vi "C3 to Cube and Switch.vi"(8 "Command Info In":T1, 10 "Block Inputs":T5, 11 "Starting Position":T4) -> (0 "Command Info Out":T1)   [LabVIEW 2017]
uses:
  <vilib>/Rock Robotics/WPI/Framework/Command Status Info.ctl
  <vilib>/Rock Robotics/WPI/Framework/Completion Status.ctl
  <vilib>/Rock Robotics/WPI/Framework/Completion Notifier.ctl
  Block Clusters/C3 to Cube and Switch.ctl
  Support Code/Starting Position.ctl
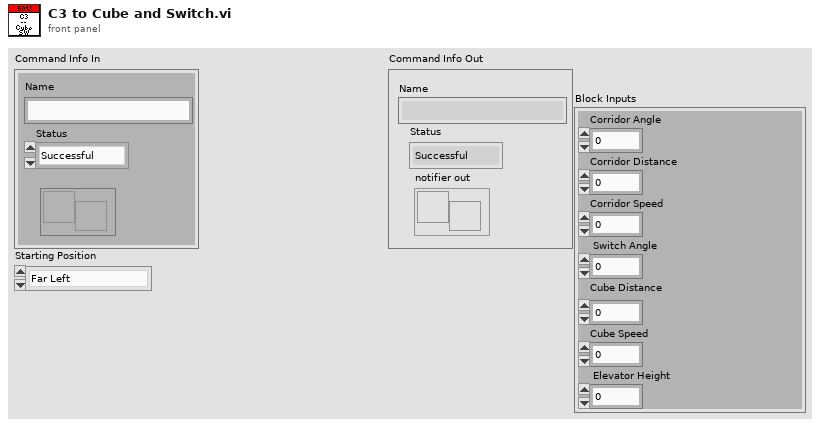
[diagram p1: front panel]
types:
  T1 = typedef "Command Status Info.ctl" = cluster{"Name":string, "Status":T2, "notifier out":T3}
  T2 = typedef "Completion Status.ctl" = enum16{"Successful", "Aborted", "Incomplete"}
  T3 = typedef "Completion Notifier.ctl" = refnum<notifier>
  T4 = typedef "Starting Position.ctl" = enum16{"Far Left", "Center", "Far Right"}
  T5 = typedef "C3 to Cube and Switch.ctl" = cluster{"Corridor Angle":dbl, "Corridor Distance":dbl, "Corridor Speed":dbl, " Switch Angle":dbl, "Cube Distance":dbl, "Cube Speed":dbl, " Elevator Height":dbl}
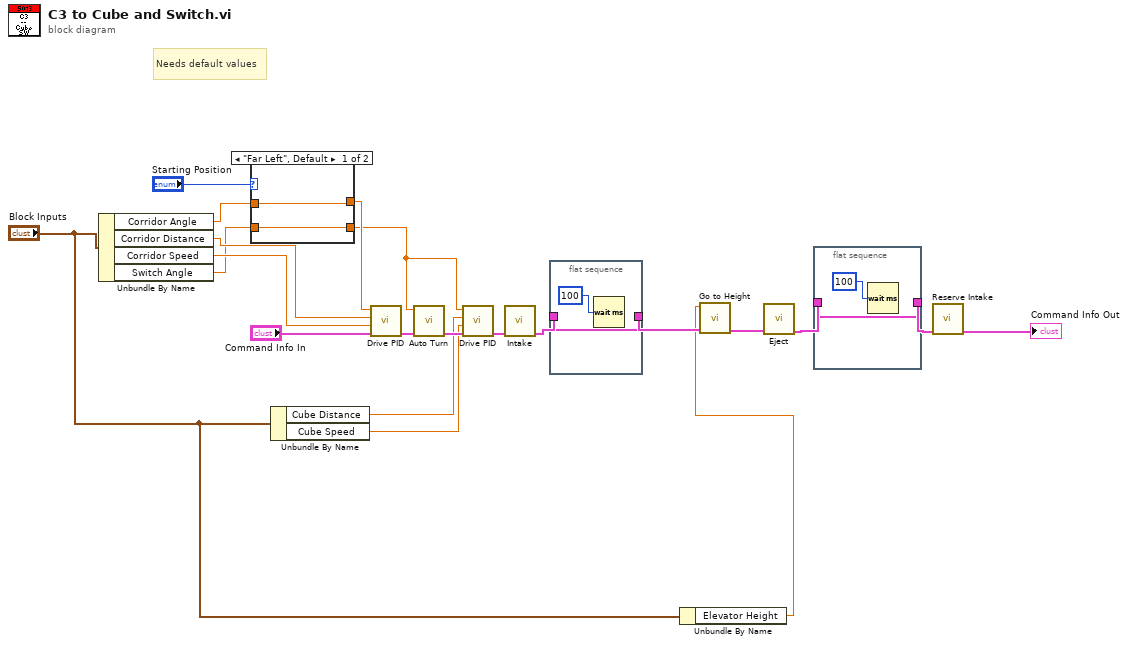
[diagram p0: block diagram]
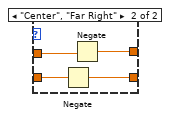
[diagram p2: hidden frame]
diagram:
  # "Needs default values"
  n1 = Unbundle By Name("Block Inputs") -> ("Corridor Angle"=w10:dbl, "Corridor Distance"=w8:dbl, "Corridor Speed"=w7:dbl, "Switch Angle"=w6:dbl)
  n2 = case shown="\"Far Left\", Default" "Starting Position" {
    tunnel: [w23 w27] -> w9
    tunnel: w10 -> [w23 w26]
    tunnel: w6 -> [w22 w25]
    tunnel: [w22 w24] -> w5
    frame "Far Left", Default {
    }
    frame "Center", "Far Right" {
      n3 = Negate(x=w25) -> (-x=w24:dbl)
      n4 = Negate(x=w26) -> (-x=w27:dbl)
    }
  }
  n5 = Unbundle By Name("Block Inputs") -> ("Cube Distance"=w4:dbl, "Cube Speed"=w3:dbl)
  n6 = call "Drive PID.vi"("Command Info In"="Command Info In", "Speed"=w7, "Distance"=w8, "Target Angle"=w9) -> ("Command Info Out"=w19:T1)  [unwired: 7 in]
  n7 = call "Auto Turn.vi"("Command Info In"=w19, "Target Angle"=w5) -> ("Command Info Out"=w18:T1)  [unwired: 9 in]
  n8 = call "Drive PID.vi"("Command Info In"=w18, "Speed"=w3, "Distance"=w4, "Target Angle"=w5) -> ("Command Info Out"=w16:T1)  [unwired: 7 in]
  n9 = call "Intake.vi"("Command Info In"=w16) -> ("Command Info Out"=w14:T1)  [unwired: 10 in]
  n10 = flat-sequence {
    tunnel: w14 -> [w29]
    tunnel: [w29] -> w13
    frame #0 {
      n11 = Wait (ms)(milliseconds to wait=u32 100) -> ()  [unwired: 1 out]
    }
  }
  n12 = Unbundle By Name("Block Inputs") -> ("Elevator Height"=w1:dbl)
  n13 = call "Go to Height.vi"("Command Info In"=w13, "Target Height (in)"=w1) -> ("Command Info Out"=w12:T1)  [unwired: 9 in]
  n14 = call "Eject.vi"("Command Info In"=w12) -> ("Command Info Out"=w15:T1)  [unwired: 10 in]
  n15 = flat-sequence {
    tunnel: w15 -> [w30]
    tunnel: [w30] -> w17
    frame #0 {
      n16 = Wait (ms)(milliseconds to wait=u32 100) -> ()  [unwired: 1 out]
    }
  }
  n17 = call "Reserve Intake.vi"("Command Info"=w17) -> ("Command Info"=→"Command Info Out":T1)  [unwired: 10 in]
